vi "SIPO_Present_CLR.vi"(4 "Clear":bool, 5 "Frequency":dbl, 6 "Serial":bool) -> (0 "Q4":bool, 1 "Q3":bool, 2 "Q2":bool, 3 "Q1":bool)   [LabVIEW 2018]
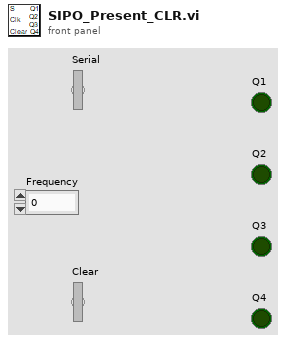
[diagram p1: front panel]
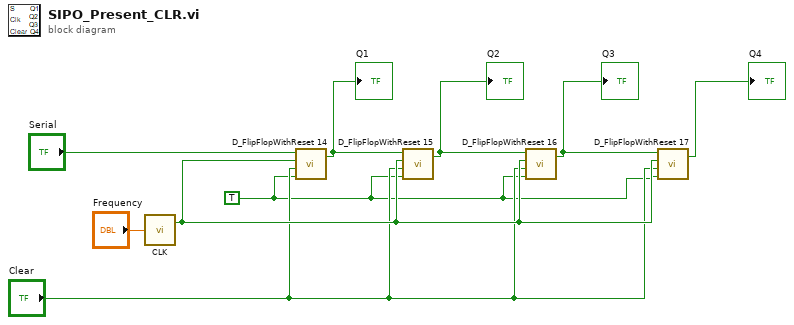
[diagram p0: block diagram]
diagram:
  w1 = TRUE
  n1 = call "CLK.vi"("Frequency"="Frequency") -> ("CLK"=w3:bool)  [unwired: 1 out]
  n2 = call "D_FlipFlopWithReset 14.vi"("________\nPresent"=w1, "______\nClear"="Clear", "CLK"=w3, "D"="Serial") -> ("Q"=w8:bool)  [unwired: 1 out]
  "Q1" <- w8
  n3 = call "D_FlipFlopWithReset 15.vi"("________\nPresent"=w1, "______\nClear"="Clear", "CLK"=w3, "D"=w8) -> ("Q"=w7:bool)  [unwired: 1 out]
  "Q2" <- w7
  n4 = call "D_FlipFlopWithReset 16.vi"("________\nPresent"=w1, "______\nClear"="Clear", "CLK"=w3, "D"=w7) -> ("Q"=w5:bool)  [unwired: 1 out]
  "Q3" <- w5
  n5 = call "D_FlipFlopWithReset 17.vi"("________\nPresent"=w1, "______\nClear"="Clear", "CLK"=w3, "D"=w5) -> ("Q"=→"Q4":bool)  [unwired: 1 out]
